vi "Configure Segment.vi"(0 "VISA resource name":refnum<visa-resource-name>, 1 "IF Bandwidth (20k Hz)":dbl=20000.0, 2 "Sweep Time (1 s)":dbl=1.0, 5 "Channel (1)":i32=1, 7 "Segment Number (1)":i32=1, 9 "Enable Segment (F: Disable)":bool, 11 "error in (no error)":errorcluster, 12 "Number of Points (21)":i32=21) -> (4 "VISA resource name out":refnum<visa-resource-name>, 15 "error out":errorcluster)   [LabVIEW 2018, in "Keysight PNA Series.lvlib"]
doc: "Configures segment sweep."
uses:
  Keysight PNA Series.lvlib
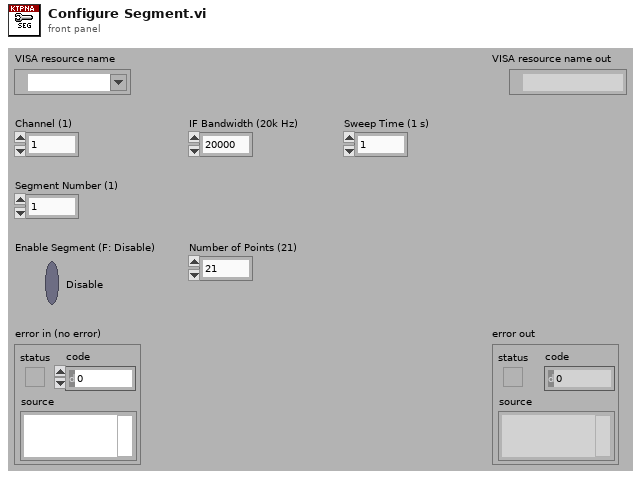
[diagram p1: front panel]
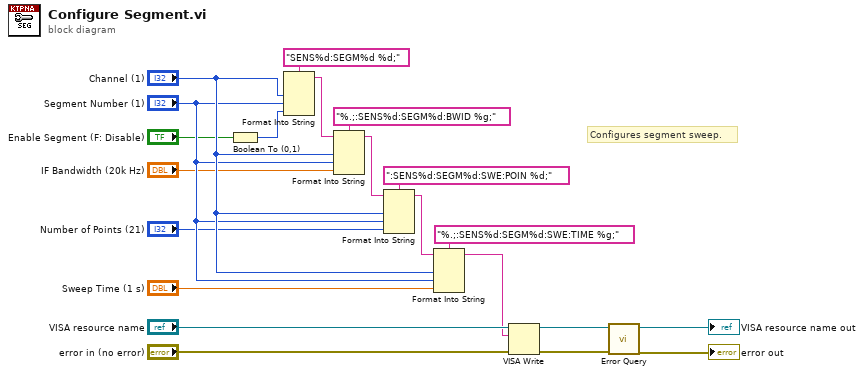
[diagram p0: block diagram]
diagram:
  # "Configures segment sweep."
  n1 = Boolean To (0,1)(Boolean="Enable Segment (F: Disable)") -> (0, 1=w3:i16)
  n2 = Format Into String(format string="SENS%d:SEGM%d %d;", "Channel (1)", "Segment Number (1)", w3) -> (resulting string=w18:string)  [unwired: 2 in, 1 out]
  n3 = Format Into String(format string="%.;:SENS%d:SEGM%d:BWID %g;", initial string=w18, "Channel (1)", "Segment Number (1)", "IF Bandwidth (20k Hz)") -> (resulting string=w2:string)  [unwired: 1 in, 1 out]
  n4 = Format Into String(format string=":SENS%d:SEGM%d:SWE:POIN %d;", initial string=w2, "Channel (1)", "Segment Number (1)", "Number of Points (21)") -> (resulting string=w13:string)  [unwired: 1 in, 1 out]
  n5 = Format Into String(format string="%.;:SENS%d:SEGM%d:SWE:TIME %g;", initial string=w13, "Channel (1)", "Segment Number (1)", "Sweep Time (1 s)") -> (resulting string=w1:string)  [unwired: 1 in, 1 out]
  n6 = VISA Write(VISA resource name="VISA resource name", write buffer=w1, error in (no error)="error in (no error)") -> (VISA resource name out=w8:refnum<visa-resource-name>, error out=w7:errorcluster)  [unwired: 1 out]
  n7 = call "Error Query.vi"("error in (no error)"=w7, "VISA resource name"=w8) -> ("error out"=→"error out":errorcluster, "VISA resource name out"=→"VISA resource name out":refnum<visa-resource-name>)  [unwired: 6 in, 2 out]
